vi "Pre Launch Init.vi"(11 "RDS Logger Actor in":refnum<class "RDS Logger Actor.lvclass">) -> (0 "error out":errorcluster, 3 "RDS Logger Actor out":refnum<class "RDS Logger Actor.lvclass">)   [LabVIEW 2015, in "RDS Logger Actor.lvlib" / "RDS Logger Actor.lvclass"]
doc: "Sends a high priority message to it's self to notify the monitor that it's spawned. If it's in the runtime environment, this message is never sent, meaning the monitor will never spawn\n\nCopyright: MGI\n\nAuthored by Derek Trepanier\nsupport@mooregoodideas.com\nwww.mooregoodideas.com\n\nCopyright (c) 2014, Moore Good Ideas, Inc.\n\nAll rights reserved.\n\nRedistribution and use in source and binary forms, with or without modification, are permitted provided that the following conditions are met:\n\n * Redistributions of source code must retain the above copyright notice, this list of conditions and the following disclaimer.\n * Redistributions in binary form must reproduce the above copyright notice, this list of conditions and the following disclaimer in the documentation and/or other materials provided with the distribution.\n * Neither the name of Moore Good Ideas, Inc. nor the names of its contributors may be used to endorse or promote products derived from this software without specific prior written permission.\n\nTHIS SOFTWARE IS PROVIDED BY THE COPYRIGHT HOLDERS AND CONTRIBUTORS \"AS IS\" AND ANY EXPRESS OR IMPLIED WARRANTIES, INCLUDING, BUT NOT LIMITED TO, THE IMPLIED WARRANTIES OF MERCHANTABILITY AND FITNESS FOR A PARTICULAR PURPOSE ARE DISCLAIMED. IN NO EVENT SHALL THE COPYRIGHT OWNER OR CONTRIBUTORS BE LIABLE FOR ANY DIRECT, INDIRECT, INCIDENTAL, SPECIAL, EXEMPLARY, OR CONSEQUENTIAL DAMAGES (INCLUDING, BUT NOT LIMITED TO, PROCUREMENT OF SUBSTITUTE GOODS OR SERVICES; LOSS OF USE, DATA, OR PROFITS; OR BUSINESS INTERRUPTION) HOWEVER CAUSED AND ON ANY THEORY OF LIABILITY, WHETHER IN CONTRACT, STRICT LIABILITY, OR TORT (INCLUDING NEGLIGENCE OR OTHERWISE) ARISING IN ANY WAY OUT OF THE USE OF THIS SOFTWARE, EVEN IF ADVISED OF THE POSSIBILITY OF SUCH DAMAGE."
uses:
  RDS Logger Actor.lvclass
  Logger Header.ctl
  RDS Logger Actor.lvclass/RDS Logger Actor.ctl
  RDS Parent Actor/RDS Parent Actor/RDS Parent Actor.lvclass
  Libraries/Configuration Library/RDS Configuration Library.lvlib
  Utilities/Log/Log Waveform Processors.lvlib
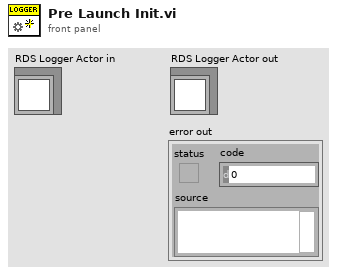
[diagram p1: front panel]
types:
  T1 = typedef "Log Waveform Processors.lvlib/Logger Header.ctl" = cluster{"Start Time":timestamp, "Update Rate (Hz)":dbl}
  T2 = enum16{"open", "replace", "create", "open or create", "replace or create", "replace or create with confirmation"}
  T3 = typedef "RDS Configuration Library.lvlib/RDS Configuration.ctl" = cluster{"State Update Rate (Hz)":dbl, "Helm Rate (Hz)":dbl, "Helm Gains":T4, "Limiter":dbl, "Mission Controller Settings":T5, "Mag Dev":dbl}
  T4 = typedef "RDS Child Messages.lvlib/PID Gains Control.ctl" = cluster{"P (Kc)":sgl, "I (Ti)":sgl, "D (Td)":sgl}
  T5 = typedef "RDS Mission Controller Actor.lvlib/Mission Controller Settings.ctl" = cluster{"Waypoint Radius (m)":dbl}
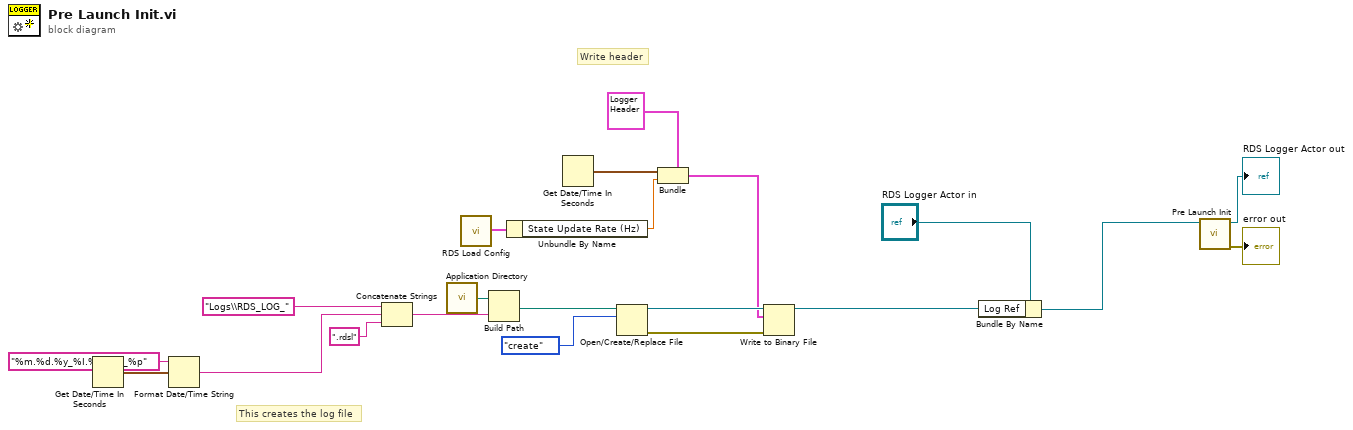
[diagram p0: block diagram]
diagram:
  # "Write header"
  # "This creates the log file"
  n1 = Get Date/Time In Seconds() -> (seconds since 1Jan1904=w16:timestamp)
  n2 = Format Date/Time String(time format string (%c)="%m.%d.%y_%I.%M.%S_%p", seconds (now)=w16) -> (date/time string=w15:string)  [unwired: 1 in]
  n3 = Concatenate Strings("Logs\\RDS_LOG_" ("name or relative path"), w15, ".rdsl" ("string")) -> (w12:string)
  n4 = call <vilib>:"Application Directory.vi"() -> ("Application Directory"=w17:path)
  n5 = call "RDS Load Config.vi"() -> ("RDS Config"=w6:T3)  [unwired: 11 in]
  n6 = Build Path(base path=w17, name or relative path=w12) -> (appended path=w11:path)
  n7 = Unbundle By Name(w6) -> ("State Update Rate (Hz)"=w4:dbl)
  n8 = Get Date/Time In Seconds() -> (seconds since 1Jan1904=w5:timestamp)
  n9 = Open/Create/Replace File(file path (use dialog)=w11, operation (0:open)=T2."create") -> (refnum out=w8:refnum<file>, error out=w1:errorcluster)  [unwired: 4 in, 1 out]
  n10 = Bundle(cluster=T1 {"Start Time"=timestamp(0 s since 1904-01-01), "Update Rate (Hz)"=0.0} ("Log Header"), "Start Time"=w5, "Update Rate (Hz)"=w4) -> (w2:T1)
  n11 = Write to Binary File(file (use dialog)=w8, data=w2, error in=w1) -> (refnum out=w7:refnum<file>)  [unwired: 3 in, 2 out]
  n12 = Bundle By Name(cluster="RDS Logger Actor in", "Log Ref"=w7) -> (w18:refnum<class "RDS Logger Actor.lvclass">)
  n13 = call-parent "Pre Launch Init.vi"("Actor in"=w18) -> ("error out"=→"error out":errorcluster, "Actor out"=→"RDS Logger Actor out":refnum<class "RDS Logger Actor.lvclass">)  [unwired: 9 in]
